vi "VS_GetStimProfileState_TS_Step.vi"(0 "Engine reference":refnum<k7>, 5 "Sequence File Ref":refnum<k7>, 7 "Step Name":string="Open Workspace Manager Reference", 9 "Parameter Value array":string[](array[string])=["Locals.StimState"], 11 "error in":errorcluster, 12 "Sequence index":i32, 13 "RecordResult":bool=TRUE, 14 "Precondition":string) -> (4 "Engine reference (out)":refnum<k7>, 6 "Sequence File Ref(out)":refnum<k7>, 15 "error out":errorcluster)   [LabVIEW 2010]
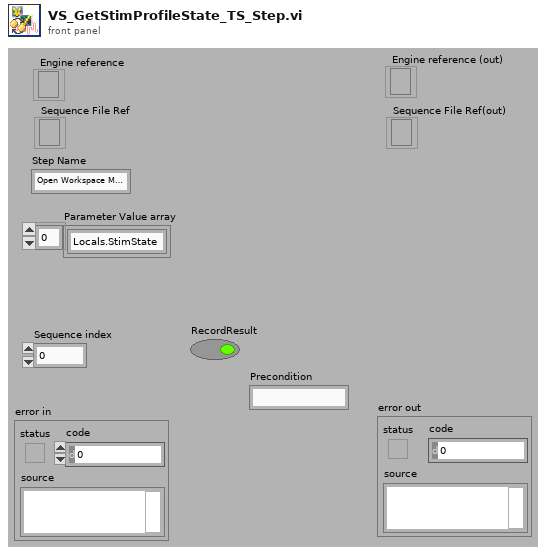
[diagram p1: front panel]
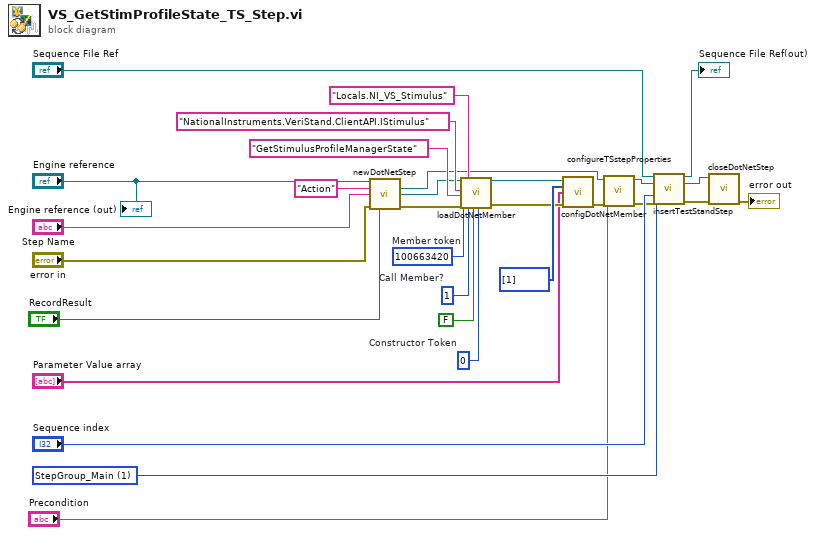
[diagram p0: block diagram]
diagram:
  w28 = 100663420  # Member token
  w26 = 1 items=["StepGroup_Setup", "StepGroup_Main", "StepGroup_Cleanup"] ("Step Group")
  w23 = 0  # Constructor Token
  w21 = 1  # Call Member?
  n1 = call "newDotNetStep.vi"("Engine reference"="Engine reference", "stepType"="Action", "Step Name"="Step Name", "error in"="error in", "RecordResult"="RecordResult") -> ("NewStep (out)"=w4:refnum<k7>, "dotNetModule(out)"=w18:refnum<k7>, "error out"=w29:errorcluster)  [unwired: 7 in, 1 out]
  n2 = call "loadDotNetMember.vi"("dotNetModule"=w18, "ClassName"="NationalInstruments.VeriStand.ClientAPI.IStimulus", "MemberName"="GetStimulusProfileManagerState", "Member token"=w28, "error in(no error)"=w29, "ClassReference"="Locals.NI_VS_Stimulus", "Call Member?"=w21, "CreateObject"=FALSE, "Constructor Token"=w23) -> ("dotNetModule(out)"=w24:refnum<k7>, "error out"=w25:errorcluster)  [unwired: 9 in]
  n3 = call "configDotNetMember.vi"("dotNetModule"=w24, "Index array"=i32[] [1], "Parameter Value array"="Parameter Value array", "error in (no error)"=w25) -> ("error out"=w5:errorcluster)  [unwired: 11 in]
  n4 = call "configureTSstepProperties.vi"("error in"=w5, "Precondition"="Precondition", "NewStep (in)"=w4) -> ("error out"=w2:errorcluster, "NewStep (out)"=w3:refnum<k7>)  [unwired: 7 in]
  n5 = call "insertTestStandStep.vi"("Sequence File Ref"="Sequence File Ref", "Step to insert"=w3, "Step Group"=w26, "index"="Sequence index", "error out"=w2) -> ("Sequence File Ref(out)"=→"Sequence File Ref(out)":refnum<k7>, "Step to insert (out)"=w15:refnum<k7>, "error out"=w14:errorcluster)  [unwired: 8 in]
  n6 = call "closeDotNetStep.vi"("error in"=w14, "NewStep"=w15) -> ("error out"=→"error out":errorcluster)  [unwired: 9 in]
  "Engine reference (out)" <- "Engine reference"
